vi "Camera calibration.vi"() -> ()   [LabVIEW 2023]
uses:
  <vilib>/Utility/file.llb/Read Delimited Spreadsheet (DBL).vi
panel:
  out "X Distances":dbl[](graph)
  out "X Distances":dbl[](array[numeric])
  out "subarray":dbl[](array[numeric])
  out "all rows":dbl[][](array[numeric])
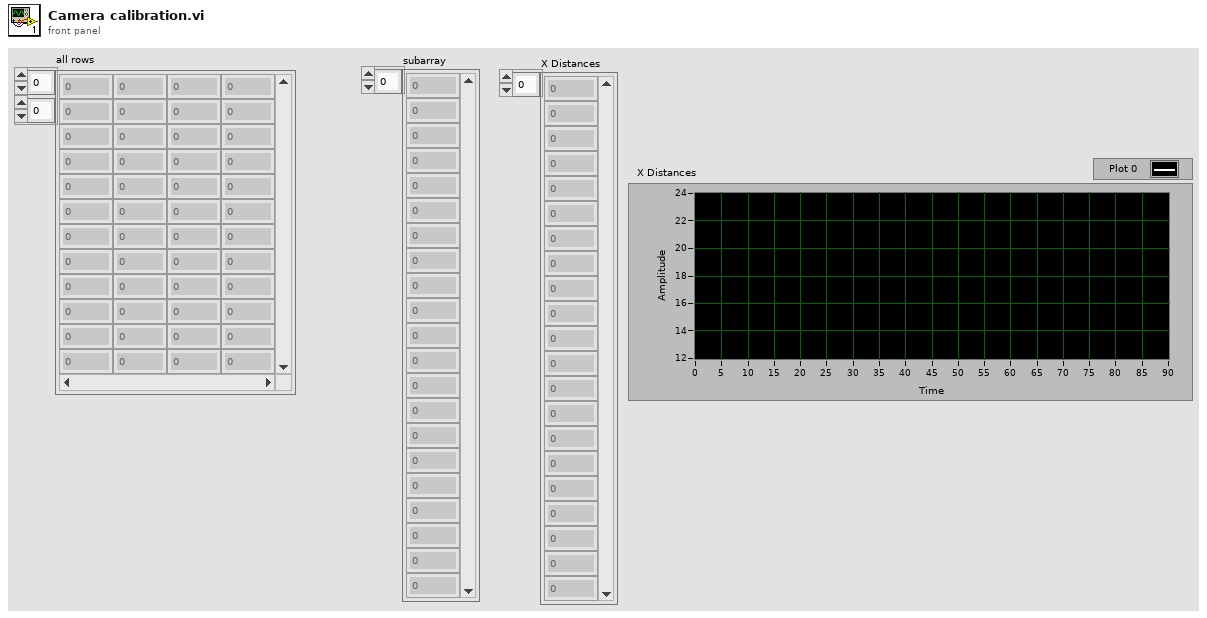
[diagram p1: front panel]
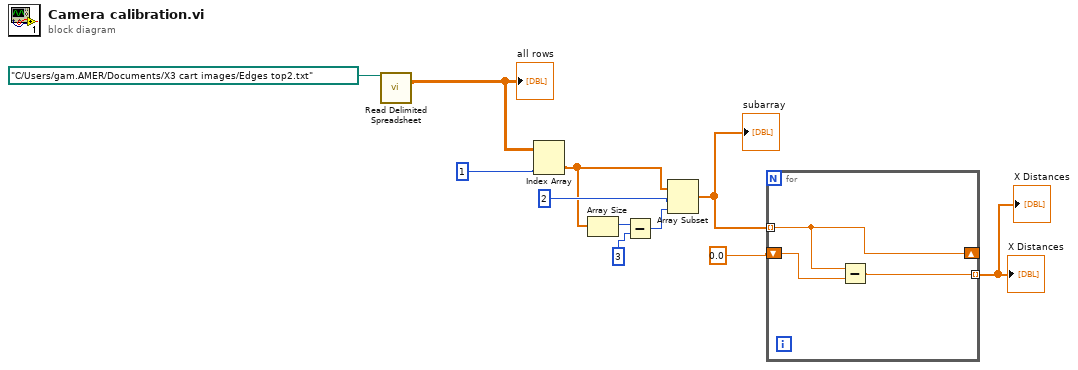
[diagram p0: block diagram]
diagram:
  n1 = call-poly <vilib>:"Read Delimited Spreadsheet.vi"("file path (dialog if empty)"=path "C:/Users/gam.AMER/Documents/X3 cart images/Edges top2.txt") -> ("all rows"=w10:dbl[][])  [unwired: 9 in, 5 out]
  "all rows" <- w10
  n2 = Index Array(array=w10, index (col)=1) -> (element=w4:dbl[])  [unwired: 1 in]
  n3 = Array Size(array=w4) -> (size(s)=w3:i32)
  n4 = Subtract(x=w3, y=3 ("index")) -> (x-y=w2:i32)
  n5 = Array Subset(array=w4, index=2, length=w2) -> (w7:dbl[])
  "subarray" <- w7
  n6 = for {
    tunnel: w7 -> [w14] mode=indexing
    shift-right: [w14] -> _
    shift-left: 0.0 ("Numeric") -> [w13]
    tunnel: [w12] -> w5 mode=indexing
    n7 = Subtract(x=w14, y=w13) -> (x-y=w12:dbl)
  }
  "X Distances" <- w5
  "X Distances" <- w5
